vi "Exhaust.vi"() -> ()   [LabVIEW 2011]
panel:
  in  "90":bool caption="49"
  in  "13":bool caption="49"
  in  "103":bool caption="49"
  out "BAR 93":dbl format="%#_5e"
  # "AsH3 1-DD VENT"
  # "AsH3 2-DD VENT"
  # "Si2H6 DD VENT"
  # "HYDRIDE VENT"
  # "ALKYL VENT"
  # "VENT"
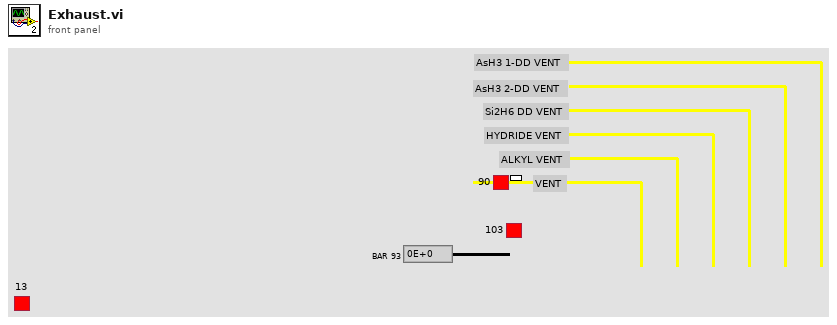
[diagram p1: front panel]
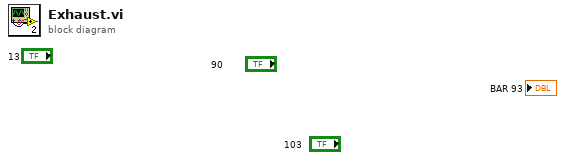
[diagram p0: block diagram]
diagram:
